vi "3D Picture_rotate_robot.vi"() -> ()   [LabVIEW 2014]
uses:
  <vilib>/Utility/miscctls.llb/LVRGBAColorTypeDef.ctl
  <vilib>/picture/3D Picture Control/Object/Create Object (name).vi
  <vilib>/picture/3D Picture Control/NI_3D Picture Control.lvlib
panel:
  in  "Specular":T1
  in  "Color Mode":T2(ring)
  in  "Ambient":T1
  in  "Scale":cluster{"X":sgl, "Y":sgl, "Z":sgl}
  in  "STL File Path":path
  in  "Yaw":dbl(knob) scale=0.0..360.0
  in  "Pitch":dbl(knob) scale=0.0..360.0
  in  "Roll":dbl(knob) scale=0.0..360.0
  in  "Stop":bool
  out "3D Picture":refnum<vi>(3d-picture)
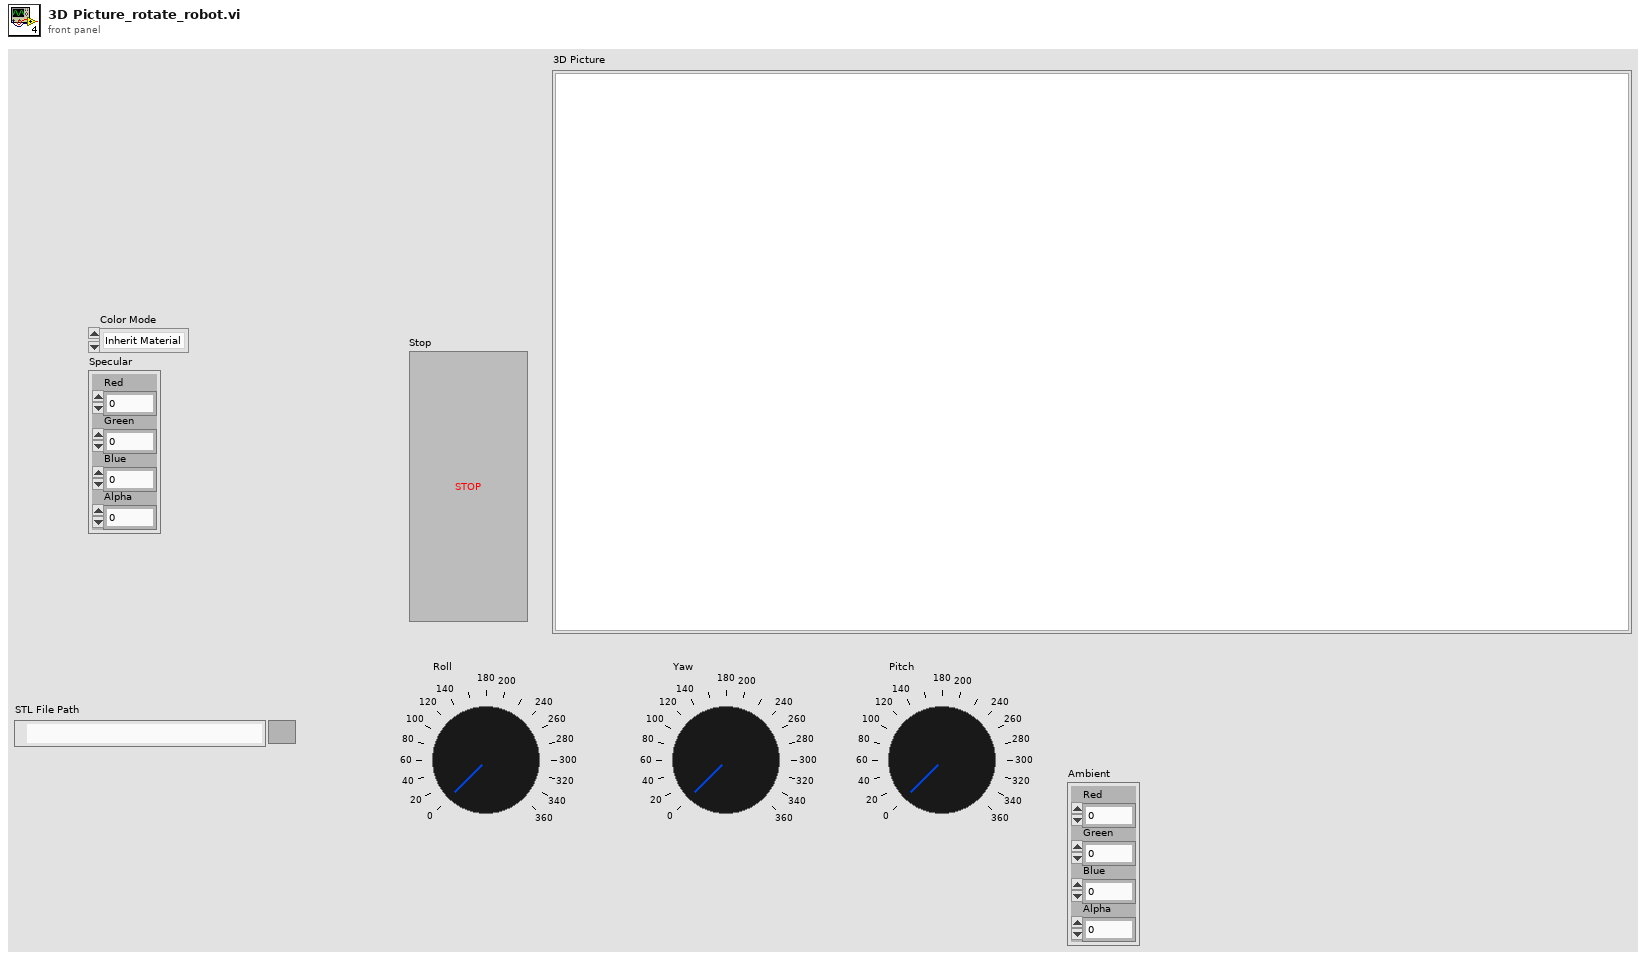
[diagram p1: front panel]
types:
  T1 = typedef "LVRGBAColorTypeDef.ctl" = cluster{"Red":sgl, "Green":sgl, "Blue":sgl, "Alpha":sgl}
  T2 = enum16{"Inherit Material", "Use entire Material", "Ignore Ambient", "Ignore Diffuse", "Ignore Specular", "Ignore Emission", "Ignore Ambient and Diffuse"}
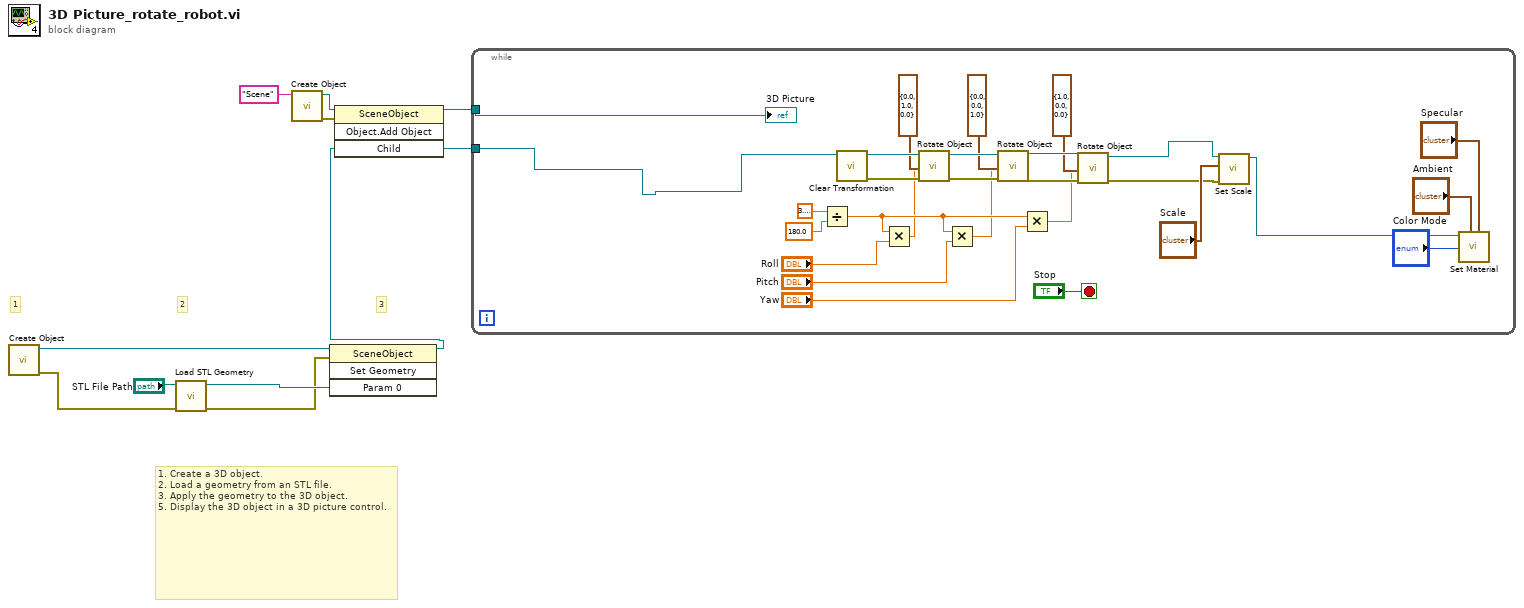
[diagram p0: block diagram]
diagram:
  # "3"
  # "2"
  # "1"
  # "1. Create a 3D object.\n2. Load a geometry from an STL file.\n3. Apply the geometry to the 3D object.\n5. Display the 3D object in a 3D picture control."
  n1 = call-poly <vilib>:"Create Object.vi"() -> ("error out"=w5:errorcluster, "Scene:New Object"=w6:refnum<vi>)  [unwired: 10 in]
  n2 = call <vilib>:"Load STL Geometry.vi"("error in (no error)"=w5, "Model File"="STL File Path") -> ("error out"=w3:errorcluster, "New Mesh Refnum"=w4:refnum<vi>)  [unwired: 8 out]
  n3 = call-poly <vilib>:"Create Object.vi"("Name"="Scene") -> ("error out"=w11:errorcluster, "Scene:New Object"=w10:refnum<vi>)  [unwired: 9 in]
  n4 = invoke class="SceneObject" method="Set Geometry"(reference=w6, error in=w3, "Param 0"=w4) -> (reference out=w1:refnum<vi>)  [unwired: 1 in, 3 out]
  n5 = invoke class="SceneObject" method="Object.Add Object"(reference=w10, error in=w11, "Child"=w1) -> (reference out=w8:refnum<vi>, "Child"=w2:refnum<vi>)  [unwired: 1 in, 2 out]
  n6 = while {
    tunnel: w8 -> [w13]
    tunnel: w2 -> [w12]
    stop <- "Stop" stop-if-true
    n7 = Divide(x=3.141592653589793, y=180.0) -> (x/y=w28:dbl)
    n8 = call <vilib>:"Clear Transformation.vi"("Object Refnum In"=w12) -> ("error out"=w36:errorcluster, "Object Refnum Out"=w37:refnum<vi>)  [unwired: 9 in]
    n9 = Multiply(x=w28, y="Roll") -> (x*y=w25:dbl)
    n10 = call <vilib>:"Rotate Object.vi"("error in (no error)"=w36, "Angle"=w25, "Axis"=cluster{"X":sgl, "Y":sgl, "Z":sgl} {"X"=0.0, "Y"=1.0, "Z"=0.0}, "Scene.Object In"=w37) -> ("error out"=w38:errorcluster, "Scene.Object Out"=w39:refnum<vi>)  [unwired: 6 in]
    n11 = Multiply(x=w28, y="Pitch") -> (x*y=w24:dbl)
    n12 = call <vilib>:"Rotate Object.vi"("error in (no error)"=w38, "Angle"=w24, "Axis"=cluster{"X":sgl, "Y":sgl, "Z":sgl} {"X"=0.0, "Y"=0.0, "Z"=1.0}, "Scene.Object In"=w39) -> ("error out"=w31:errorcluster, "Scene.Object Out"=w32:refnum<vi>)  [unwired: 6 in]
    n13 = Multiply(x=w28, y="Yaw") -> (x*y=w27:dbl)
    n14 = call <vilib>:"Rotate Object.vi"("error in (no error)"=w31, "Angle"=w27, "Axis"=cluster{"X":sgl, "Y":sgl, "Z":sgl} {"X"=1.0, "Y"=0.0, "Z"=0.0}, "Scene.Object In"=w32) -> ("error out"=w18:errorcluster, "Scene.Object Out"=w20:refnum<vi>)  [unwired: 6 in]
    n15 = call <vilib>:"Set Scale.vi"("error in (no error)"=w18, "Scale"="Scale", "Scene Object"=w20) -> ("Scaled Object"=w16:refnum<vi>)  [unwired: 7 in, 1 out]
    n16 = call <vilib>:"Set Material.vi"("Specular"="Specular", "Ambient"="Ambient", "Color Mode"="Color Mode", "Scene Object In"=w16) -> ()  [unwired: 6 in, 2 out]
    "3D Picture" <- w13
  }
